vi "BME_DG_Initialize.vi"(7 "error in (no error)":errorcluster, 8 "Slot Number":i32, 9 "DG_Product":i32, 10 "DG_Number":i32) -> (0 "error out":errorcluster, 3 "return code":i32)   [LabVIEW 2009, in "POLARIS BME DG.lvlib"]
uses:
  POLARIS BME DG.lvlib
  BME DLL/DelayGenerator.dll
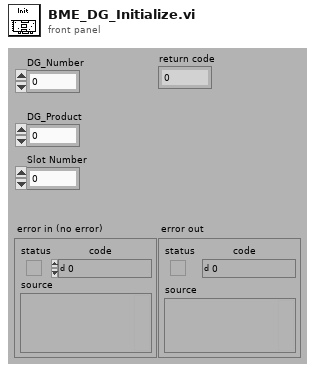
[diagram p1: front panel]
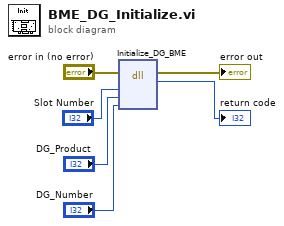
[diagram p0: block diagram]
diagram:
  n1 = dll-call lib="C:/CS Framework/LVSCC/LV2009/GPL/Projects/cs-framework/CSClass/CSPOLARIS/POLARIS BME DG/BME DLL/DelayGenerator.dll" fn="Initialize_DG_BME"(error in="error in (no error)", "base"="Slot Number", "Product"="DG_Product", "DG_Number"="DG_Number") -> (error out=→"error out":errorcluster, →"return code":i32)  [unwired: 5 in, 1 out]
